vi "17-xPosToVel.vi"(1 "x position":dbl) -> (0 "x velocity":dbl)   [LabVIEW 2019, in "17.lvlib"]
uses:
  17.lvlib
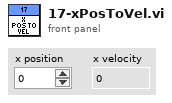
[diagram p1: front panel]
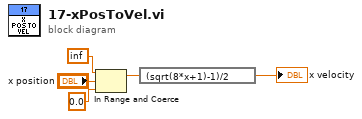
[diagram p0: block diagram]
diagram:
  n1 = In Range and Coerce(upper limit=inf, x="x position", lower limit=0.0 ("upper limit")) -> (coerced(x)=w4:dbl)  [unwired: 1 out]
  n2 = expression code="(sqrt(8*x+1)-1)/2"(w4) -> (→"x velocity":dbl)
